vi "Write msec between samples.vi"(4 "Error In":errorcluster, 6 "msec between samples":i32, 7 "Set Acquisition Rate in":refnum<class "Remote Access Commands_Set Acquisition Rate.lvclass">) -> (0 "Error Out":errorcluster, 3 "Set Acquisition Rate out":refnum<class "Remote Access Commands_Set Acquisition Rate.lvclass">)   [LabVIEW 2015, in "Startup Processes.lvlib" / "Remote Access Commands_Set Acquisition Rate.lvclass"]
uses:
  Remote Access Commands_Set Acquisition Rate.lvclass
  Remote Access Commands_Set Acquisition Rate.lvclass/Remote Access Commands_Set Acquisition Rate.ctl
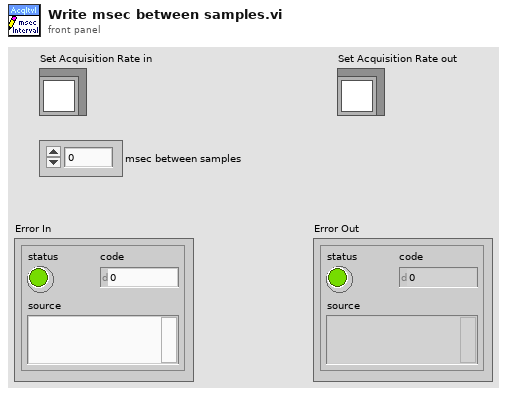
[diagram p1: front panel]
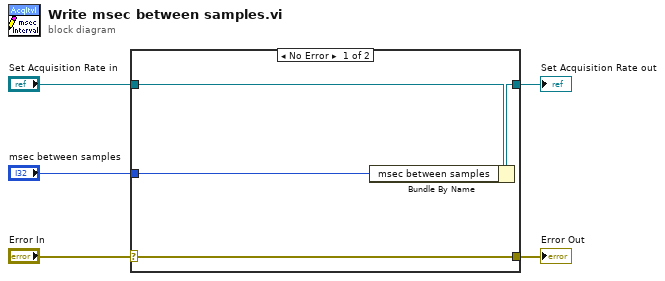
[diagram p0: block diagram]
diagram:
  n1 = case shown="No Error" "Error In" {
    selector: "Error In" -> [w9 w10]
    tunnel: [w9 w10] -> w4
    tunnel: [w7 w11] -> w2
    tunnel: "Set Acquisition Rate in" -> [w8 w11]
    tunnel: "msec between samples" -> [w6 _]
    frame No Error {
      n2 = Bundle By Name(cluster=w8, "msec between samples"=w6) -> (w7:refnum<class "Remote Access Commands_Set Acquisition Rate.lvclass">)
    }
    frame Error {
    }
  }
  "Error Out" <- w4
  "Set Acquisition Rate out" <- w2
